vi "GSP_CF_Global.vi"() -> ()   [LabVIEW 2015]
uses:
  SystemUtil/MotorStates.ctl
  SystemUtil/ThreadStates.ctl
panel:
  out "Piezo Flexure Active":bool
  in  "CF Thread State":T1
  in  "Tilt":dbl
  in  "A2":dbl
  in  "A1":dbl
  in  "Right Piezo":i32
  in  "Left Piezo":i32
  in  "CF Ext Temp":dbl
  in  "CF Motor State":T2
  in  "CF CPU Temp":dbl
  out "CF Online":bool
  in  "Position":i32
  in  "Target":i32
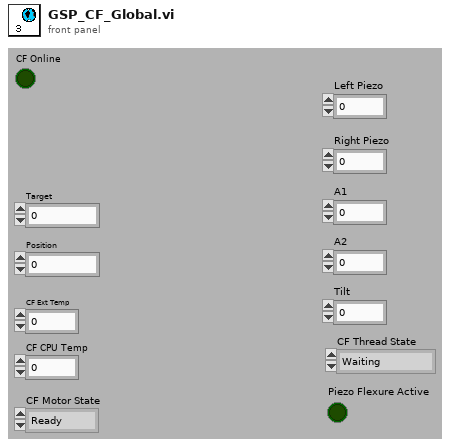
[diagram p1: front panel]
types:
  T1 = typedef "ThreadStates.ctl" = enum16{"Waiting", "Scripting", "Uninitialized", "Error"}
  T2 = typedef "MotorStates.ctl" = enum16{"Ready", "Moving", "Uninitialized", "Error"}
diagram:
